vi "FilepathString.vi"(0 "base path":path=path "C:/Users/aspit/Git/MHDLab/Test Data", 1 "Project":string, 2 "Measurement number":i32, 3 "Extra":string, 4 "Instrument":string="UnknownInst") -> (5 "Folder":path, 6 "Filename":string="Spectrometer_Run1.tdms")   [LabVIEW 2018]
uses:
  <vilib>/regexp/Match Regular Expression.xnode
panel:
  out "Month":string="5"
  out "Year":string="2018"
  out "Day":string="27"
  out "date string":string="5/27/2018"
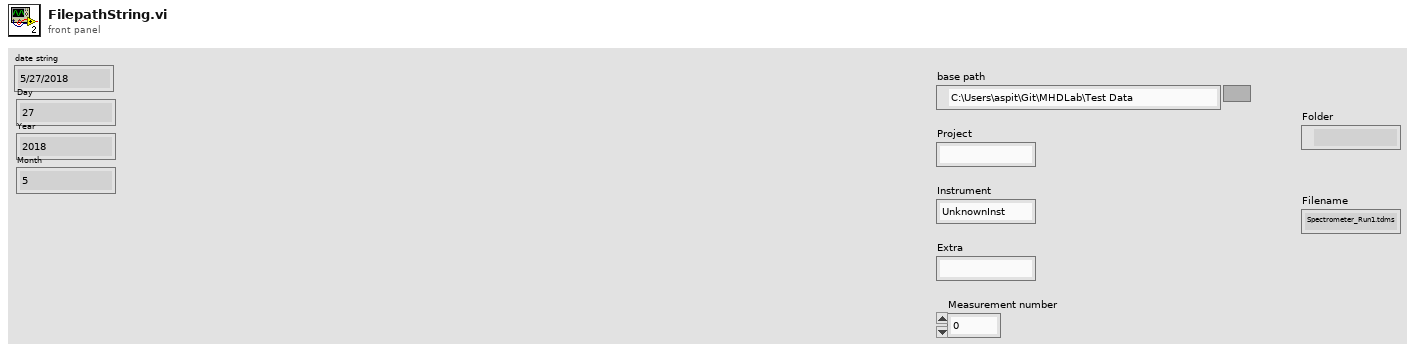
[diagram p1: front panel]
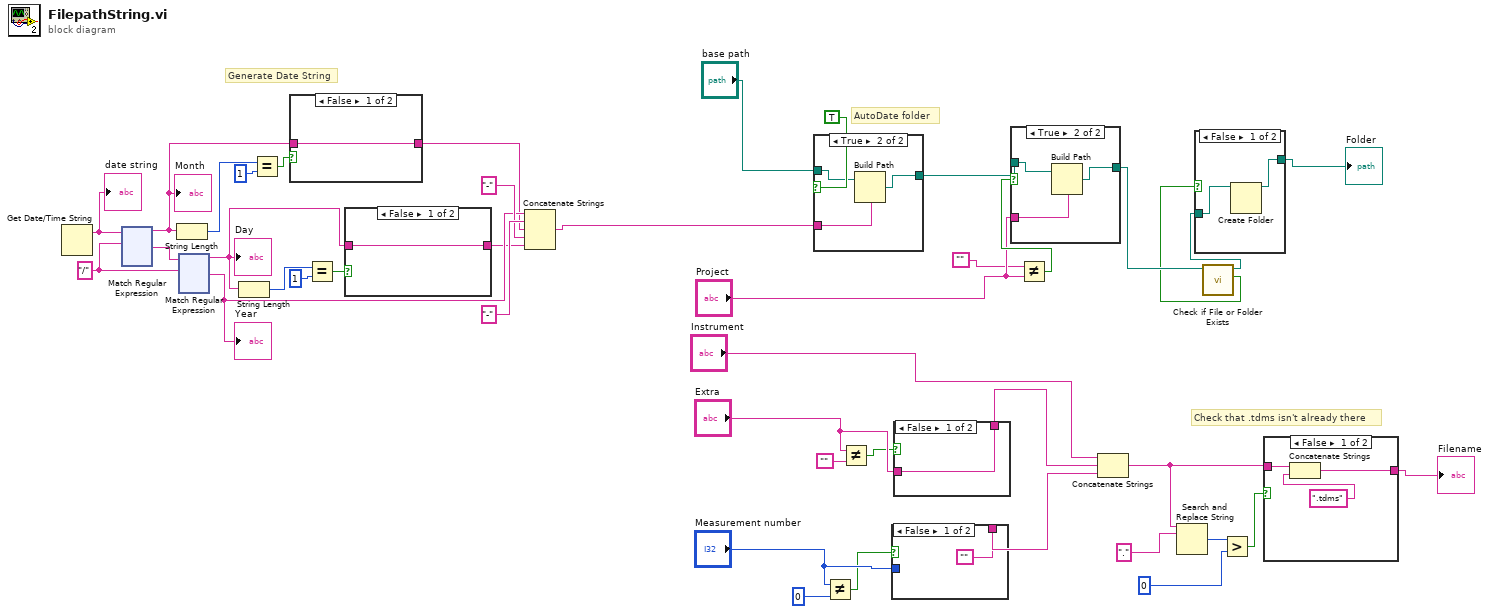
[diagram p0: block diagram]
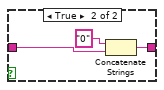
[diagram p2: hidden frame]
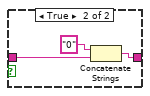
[diagram p3: hidden frame]
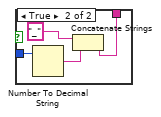
[diagram p4: hidden frame]
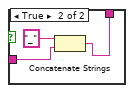
[diagram p5: hidden frame]
diagram:
  w16 = "/" ("regular expression")
  # "Generate Date String"
  # "Check that .tdms isn't already there"
  # "AutoDate folder"
  n1 = Get Date/Time String() -> (date string=w18:string)  [unwired: 3 in, 1 out]
  "date string" <- w18
  n2 = xnode "Match Regular Expression"("input string"=w18, "regular expression"=w16) -> ("before match"=w9:string, "after match"=w17:string)  [unwired: 4 in, 3 out]
  "Month" <- w9
  n3 = String Length(string=w9) -> (length=w12:i32)
  n4 = xnode "Match Regular Expression"("input string"=w17, "regular expression"=w16) -> ("before match"=w4:string, "after match"=w13:string)  [unwired: 4 in, 3 out]
  "Day" <- w4
  "Year" <- w13
  n5 = String Length(string=w4) -> (length=w5:i32)
  n6 = Equal?(x=w12, y=1) -> (x = y?=w10:bool)
  n7 = case shown="False" w10 {
    tunnel: w9 -> [w43 w46]
    tunnel: [w43 w44] -> w8
    frame False {
    }
    frame True {
      n8 = Concatenate Strings("0" ("string"), w46) -> (w44:string)
    }
  }
  n9 = Equal?(x=w5, y=1) -> (x = y?=w7:bool)
  n10 = case shown="False" w7 {
    tunnel: w4 -> [w47 w50]
    tunnel: [w47 w48] -> w3
    frame False {
    }
    frame True {
      n11 = Concatenate Strings("0" ("string"), w50) -> (w48:string)
    }
  }
  n12 = Concatenate Strings(w13, "-" ("string"), w8, "-" ("string"), w3) -> (w2:string)
  n13 = case shown="True" TRUE ("Auto Date folder") {
    tunnel: "base path" -> [w51 w54]
    tunnel: [w51 w52] -> w25
    tunnel: w2 -> [_ w53]
    frame False {
    }
    frame True {
      n14 = Build Path(base path=w54, name or relative path=w53) -> (appended path=w52:path)
    }
  }
  n15 = Not Equal?(x="Measurement number", y=0) -> (x != y?=w37:bool)
  n16 = Not Equal?(x="Extra", y="") -> (x != y?=w34:bool)
  n17 = case shown="False" w37 {
    tunnel: ["" w58] -> w41
    tunnel: "Measurement number" -> [_ w57]
    frame False {
    }
    frame True {
      n18 = Number To Decimal String(number=w57) -> (decimal integer string=w56:string)  [unwired: 1 in]
      n19 = Concatenate Strings("_" ("element"), w56) -> (w58:string)
    }
  }
  n20 = case shown="False" w34 {
    tunnel: "Extra" -> [w60 w62]
    tunnel: [w60 w61] -> w40
    frame False {
    }
    frame True {
      n21 = Concatenate Strings("_" ("element"), w62) -> (w61:string)
    }
  }
  n22 = Not Equal?(x="", y="Project") -> (x != y?=w28:bool)
  n23 = case shown="True" w28 {
    tunnel: w25 -> [w64 w67]
    tunnel: [w64 w65] -> w31
    tunnel: "Project" -> [_ w66]
    frame False {
    }
    frame True {
      n24 = Build Path(base path=w67, name or relative path=w66) -> (appended path=w65:path)
    }
  }
  n25 = Concatenate Strings("Instrument", w40, w41) -> (w42:string)
  n26 = Search and Replace String(input string=w42, search string=".") -> (number of replacements=w21:i32)  [unwired: 6 in, 3 out]
  n27 = call <vilib>:"Check if File or Folder Exists.vi"("path"=w31) -> ("file or folder exists?"=w29:bool, "dup path"=w30:path)  [unwired: 8 in, 1 out]
  n28 = case shown="False" w29 {
    tunnel: w30 -> [w69 w70]
    tunnel: [w68 w70] -> w1
    frame False {
      n29 = Create Folder(path (use dialog)=w69) -> (created path=w68:path)  [unwired: 2 in, 2 out]
    }
    frame True {
    }
  }
  "Folder" <- w1
  n30 = Greater?(x=w21, y=0) -> (0:w23:bool)
  n31 = case shown="False" w23 {
    tunnel: [w72 w74] -> w32
    tunnel: w42 -> [w71 w74]
    frame False {
      n32 = Concatenate Strings(w71, ".tdms" ("string")) -> (w72:string)
    }
    frame True {
    }
  }
  "Filename" <- w32
